vi "SV Data Type Backup.vi"(8 "Error In":errorcluster, 11 "Data Type - Variant":variant[](array[variant])) -> (0 "Error Out":errorcluster, 2 "Type array":string[](array[string]), 3 "no. variables":i32)   [LabVIEW 2014]
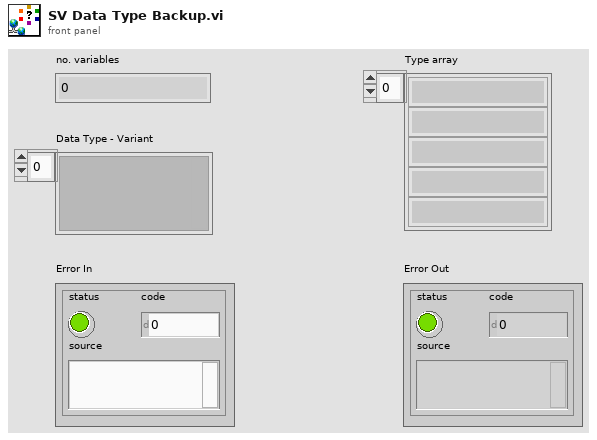
[diagram p1: front panel]
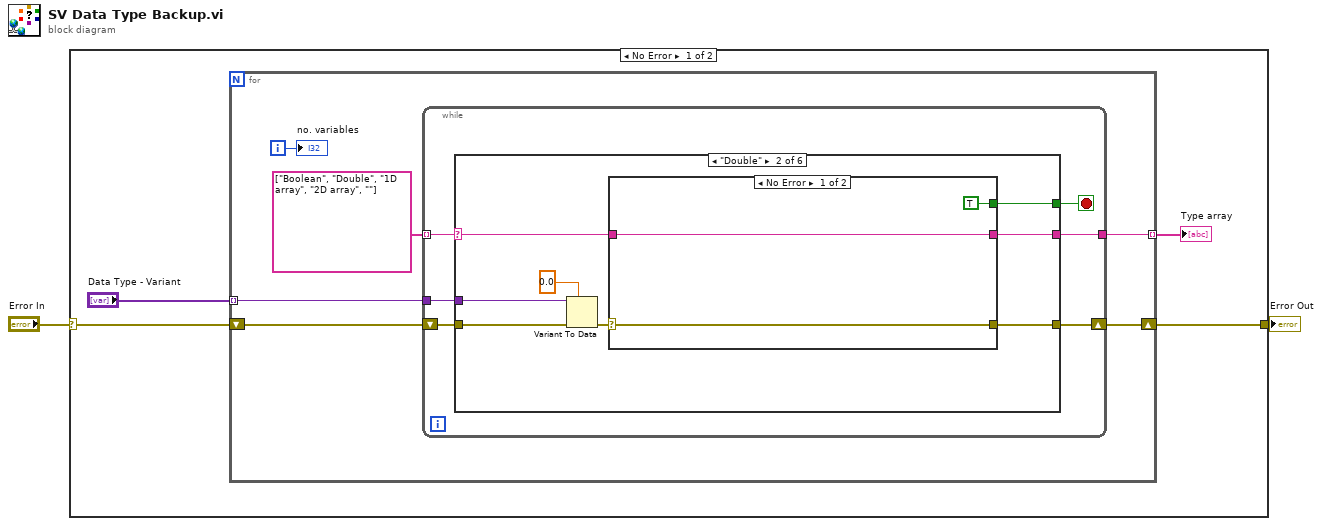
[diagram p0: block diagram]
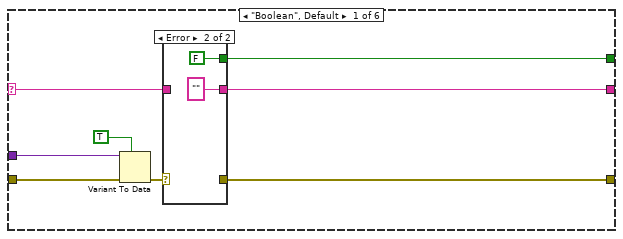
[diagram p2: hidden frame]
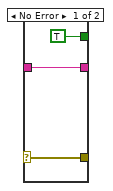
[diagram p3: hidden frame]
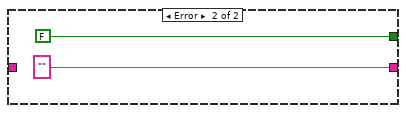
[diagram p4: hidden frame]
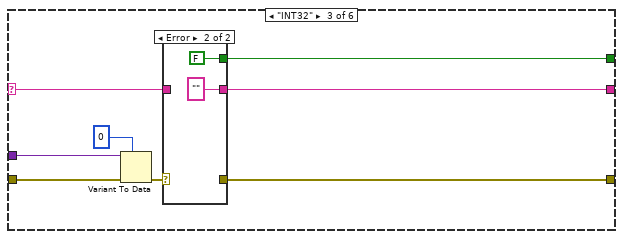
[diagram p5: hidden frame]
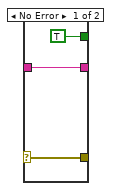
[diagram p6: hidden frame]
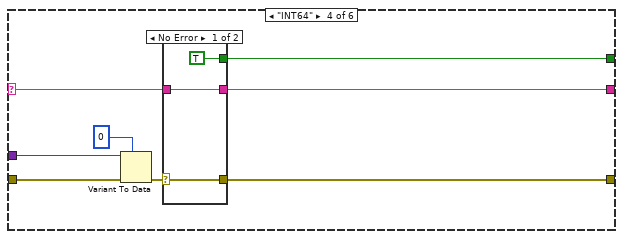
[diagram p7: hidden frame]
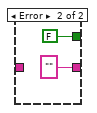
[diagram p8: hidden frame]
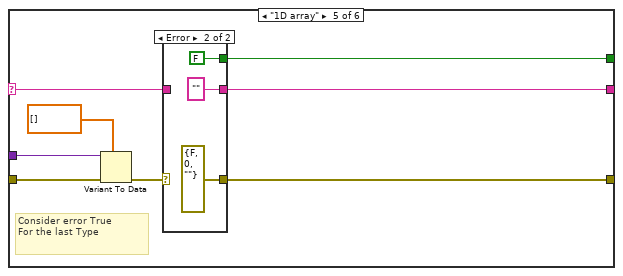
[diagram p9: hidden frame]
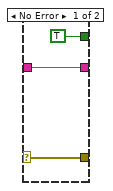
[diagram p10: hidden frame]
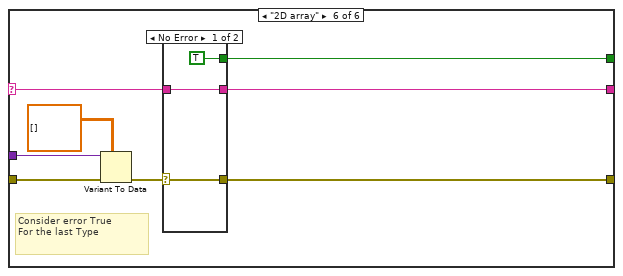
[diagram p11: hidden frame]
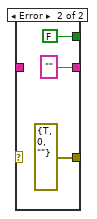
[diagram p12: hidden frame]
diagram:
  n1 = case shown="No Error" "Error In" {
    selector: "Error In" -> [w5 w99]
    tunnel: [w4 w99] -> w1
    frame No Error {
      n2 = for {
        tunnel: "Data Type - Variant" -> [w12] mode=indexing
        tunnel: [w10] -> w3 mode=indexing
        shift-right: [w7] -> w4
        shift-left: w5 -> [w8]
        i -> [w9]
        n3 = while {
          tunnel: w12 -> [w18]
          tunnel: string[] ["Boolean", "Double", "1D array", "2D array", ""] -> [w17] mode=indexing
          tunnel: [w15] -> w10
          shift-right: [w13] -> w7
          shift-left: w8 -> [w14]
          stop <- w16 stop-if-true
          n4 = case shown="\"Double\"" w17 {
            selector: w17 -> [w22 w35 w47 w62 w76 w90]
            tunnel: w18 -> [w26 w38 w50 w63 w77 w91]
            tunnel: [w23 w36 w49 w60 w74 w88] -> w16
            tunnel: [w21 w34 w48 w61 w75 w89] -> w15
            tunnel: w14 -> [w19 w33 w46 w59 w71 w85]
            tunnel: [w20 w32 w45 w58 w72 w86] -> w13
            frame "Boolean", Default {
              n5 = Variant To Data(error in=w19, type=TRUE, Variant=w26) -> (error out=w24:errorcluster)  [unwired: 1 out]
              n6 = case shown="Error" w24 {
                selector: w24 -> [w27 _]
                tunnel: [TRUE FALSE] -> w23
                tunnel: w22 -> [w28 _]
                tunnel: [w28 ""] -> w21
                tunnel: [w27 _] -> w20
                frame No Error {
                }
                frame Error {
                }
              }
            }
            frame "Double" {
              n7 = Variant To Data(error in=w33, type=0.0, Variant=w38) -> (error out=w39:errorcluster)  [unwired: 1 out]
              n8 = case shown="No Error" w39 {
                selector: w39 -> [w40 _]
                tunnel: [TRUE FALSE] -> w36
                tunnel: w35 -> [w41 _]
                tunnel: [w41 ""] -> w34
                tunnel: [w40 _] -> w32
                frame No Error {
                }
                frame Error {
                }
              }
            }
            frame "INT32" {
              n9 = Variant To Data(error in=w46, type=0, Variant=w50) -> (error out=w52:errorcluster)  [unwired: 1 out]
              n10 = case shown="Error" w52 {
                selector: w52 -> [w53 _]
                tunnel: [TRUE FALSE] -> w49
                tunnel: [w54 ""] -> w48
                tunnel: w47 -> [w54 _]
                tunnel: [w53 _] -> w45
                frame No Error {
                }
                frame Error {
                }
              }
            }
            frame "INT64" {
              n11 = Variant To Data(error in=w59, type=i64 0, Variant=w63) -> (error out=w65:errorcluster)  [unwired: 1 out]
              n12 = case shown="No Error" w65 {
                selector: w65 -> [w66 _]
                tunnel: [TRUE FALSE] -> w60
                tunnel: [w67 ""] -> w61
                tunnel: w62 -> [w67 _]
                tunnel: [w66 _] -> w58
                frame No Error {
                }
                frame Error {
                }
              }
            }
            frame "1D array" {
              # "Consider error True\nFor the last Type"
              n13 = Variant To Data(error in=w71, type=dbl[] [], Variant=w77) -> (error out=w78:errorcluster)  [unwired: 1 out]
              n14 = case shown="Error" w78 {
                selector: w78 -> [w79 _]
                tunnel: [TRUE FALSE] -> w74
                tunnel: [w80 ""] -> w75
                tunnel: w76 -> [w80 _]
                tunnel: [w79 errorcluster {"status"=FALSE, "code"=0, "source"=""} ("error IO")] -> w72
                frame No Error {
                }
                frame Error {
                }
              }
            }
            frame "2D array" {
              # "Consider error True\nFor the last Type"
              n15 = Variant To Data(error in=w85, type=dbl[][] [], Variant=w91) -> (error out=w92:errorcluster)  [unwired: 1 out]
              n16 = case shown="No Error" w92 {
                selector: w92 -> [w93 _]
                tunnel: [TRUE FALSE] -> w88
                tunnel: [w94 ""] -> w89
                tunnel: w90 -> [w94 _]
                tunnel: [w93 errorcluster {"status"=TRUE, "code"=0, "source"=""} ("error IO")] -> w86
                frame No Error {
                }
                frame Error {
                }
              }
            }
          }
        }
        "no. variables" <- w9
      }
      "Type array" <- w3
    }
    frame Error {
    }
  }
  "Error Out" <- w1
